vi "MathToolHigherOrder.vi"(0 "Time":dbl, 1 "Interp Order (NaN for Npts-1)":dbl=2.0, 2 "Data":dbl, 3 "n-int":i32 caption="points to \nintegrate over", 4 "Reset (F)":bool, 5 "n-diff":i32 caption="points to \ndifferentiate over") -> (6 "integral":dbl, 7 "1st derivative":dbl, 8 "2nd derivative":dbl)   [LabVIEW 2023]
doc: "Computes a derivative through least squares regression, a perfect interpolation, or a least coefficient norm to the provided data. If the Regression Order is unwired, the polynomial of the lowest order that perfectly interpolates the data will be used. \n\nAlso outputs the integral of P(x) over [a,b] where a and b are the first and last elements in the x array"
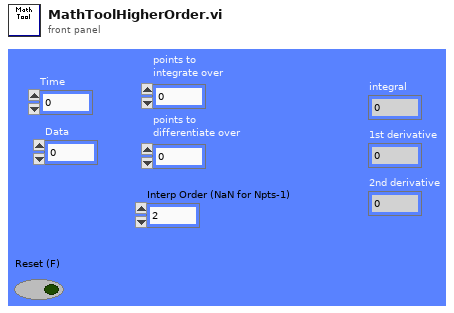
[diagram p1: front panel]
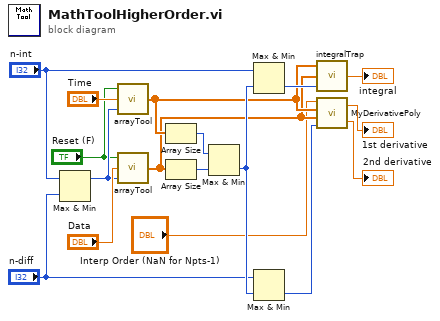
[diagram p0: block diagram]
diagram:
  n1 = Max & Min(x="n-int", y="n-diff") -> (max(x,y)=w8:i32)  [unwired: 1 out]
  n2 = call "arrayTool.vi"("Max Size"=w8, "New Element"="Time", "Reset?"="Reset (F)") -> ("Array Out"=w7:dbl[])  [unwired: 2 in]
  n3 = call "arrayTool.vi"("Max Size"=w8, "New Element"="Data", "Reset?"="Reset (F)") -> ("Array Out"=w6:dbl[])  [unwired: 2 in]
  n4 = Array Size(array=w7) -> (size(s)=w16:i32)
  n5 = Array Size(array=w6) -> (size(s)=w15:i32)
  n6 = Max & Min(x=w16, y=w15) -> (min(x,y)=w13:i32)  [unwired: 1 out]
  n7 = Max & Min(x="n-int", y=w13) -> (min(x,y)=w14:i32)  [unwired: 1 out]
  n8 = Max & Min(x="n-diff", y=w13) -> (min(x,y)=w5:i32)  [unwired: 1 out]
  n9 = call "integralTrap.vi"("n-int"=w14, "data Array"=w6, "time Array"=w7) -> ("integral"=→"integral":dbl)
  n10 = call "MyDerivativePoly.vi"("n-diff"=w5, "data Array"=w6, "time Array"=w7, "Interpolation Order"="Interp Order (NaN for Npts-1)") -> ("2nd Derivative"=→"2nd derivative":dbl, "1st Derivative"=→"1st derivative":dbl)
